vi "GetModulePic.vi"(8 "Error In":errorcluster, 11 "name":string) -> (0 "Error Out":errorcluster, 3 "new picture":picture)   [LabVIEW 2011]
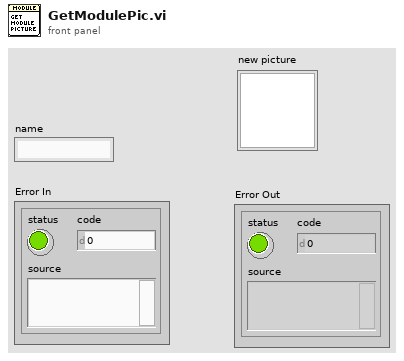
[diagram p1: front panel]
types:
  T1 = typedef "imagedata.ctl" = cluster{"image type":i32, "image depth":i32, "image":u8[], "mask":u8[], "colors":u32[], "Rectangle":cluster{"left":i16, "top":i16, "right":i16, "bottom":i16}}
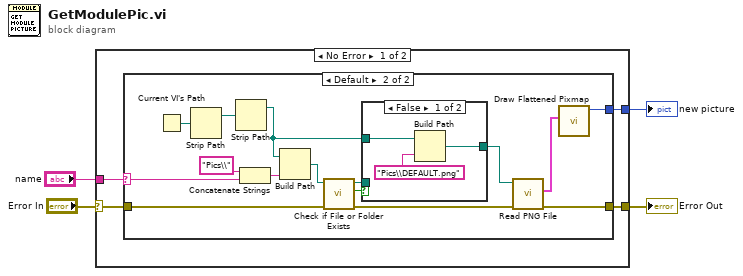
[diagram p0: block diagram]
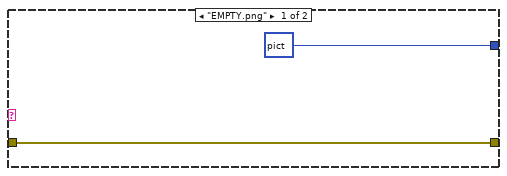
[diagram p2: hidden frame]
diagram:
  n1 = case shown="No Error" "Error In" {
    selector: "Error In" -> [w7 w30]
    tunnel: [w8 _] -> w4
    tunnel: "name" -> [w5 _]
    tunnel: [w6 w30] -> w1
    frame No Error {
      n2 = case shown="Default" w5 {
        selector: w5 -> [_ w19]
        tunnel: [picture data[5B] ("new picture") w24] -> w8
        tunnel: w7 -> [w9 w16]
        tunnel: [w9 w15] -> w6
        frame "EMPTY.png" {
        }
        frame Default {
          n3 = Current VI's Path() -> (path=w23:path)
          n4 = Strip Path(path=w23) -> (stripped path=w22:path)  [unwired: 1 out]
          n5 = Strip Path(path=w22) -> (stripped path=w11:path)  [unwired: 1 out]
          n6 = Concatenate Strings("Pics\\" ("string"), w19) -> (w20:string)
          n7 = Build Path(base path=w11, name or relative path=w20) -> (appended path=w18:path)
          n8 = call <vilib>:"Check if File or Folder Exists.vi"("error in (no error)"=w16, "path"=w18) -> ("error out"=w17:errorcluster, "file or folder exists?"=w14:bool, "dup path"=w13:path)  [unwired: 7 in]
          n9 = case shown="False" w14 {
            tunnel: w13 -> [_ w29]
            tunnel: [w26 w29] -> w12
            tunnel: w11 -> [w28 _]
            frame False {
              n10 = Build Path(base path=w28, name or relative path="Pics\\DEFAULT.png" ("string")) -> (appended path=w26:path)
            }
            frame True {
            }
          }
          n11 = call <vilib>:"Read PNG File.vi"("error in (no error)"=w17, "path to PNG file"=w12) -> ("error out"=w15:errorcluster, "image data"=w25:T1)  [unwired: 7 in, 1 out]
          n12 = call <vilib>:"Draw Flattened Pixmap.vi"("image data"=w25) -> ("new picture"=w24:picture)  [unwired: 8 in]
        }
      }
    }
    frame Error {
    }
  }
  "new picture" <- w4
  "Error Out" <- w1
